vi "Update Message.vi"(8 "error in (no error)":errorcluster, 10 "Message":string, 11 "Chat Room Controller in":refnum<class "Chat Room Controller.lvclass">) -> (0 "error out":errorcluster, 3 "Chat Room Controller out":refnum<class "Chat Room Controller.lvclass">)   [LabVIEW 2018, in "Chat Room Controller.lvlib" / "Chat Room Controller.lvclass"]
uses:
  Chat Room Controller.lvclass
  Chat Room Controller.lvclass/Chat Room Controller.ctl
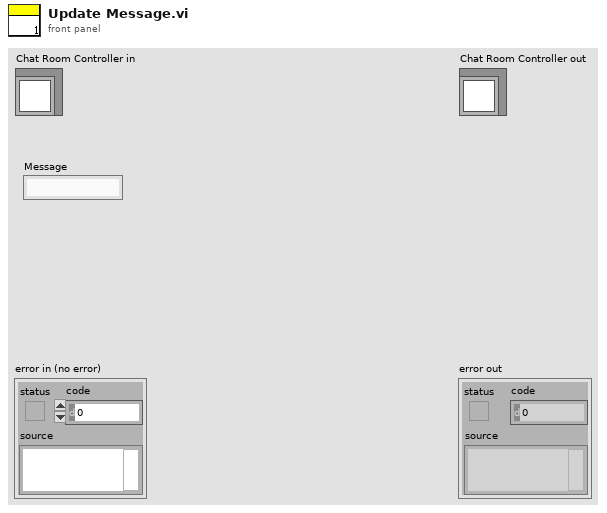
[diagram p1: front panel]
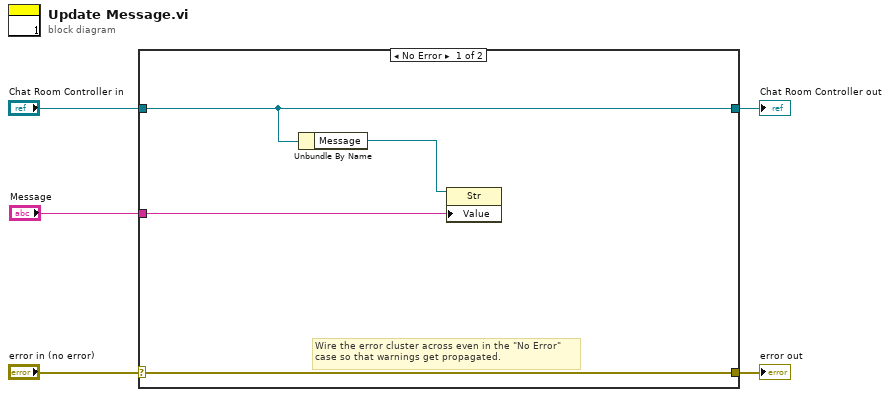
[diagram p0: block diagram]
diagram:
  n1 = case shown="No Error" "error in (no error)" {
    selector: "error in (no error)" -> [w9 w11]
    tunnel: [w9 w11] -> w4
    tunnel: [w8 w10] -> w2
    tunnel: "Chat Room Controller in" -> [w8 w10]
    tunnel: "Message" -> [w6 _]
    frame No Error {
      # "Wire the error cluster across even in the \"No Error\"\ncase so that warnings get propagated."
      n2 = Unbundle By Name(w8) -> ("Message"=w7:refnum<vi>)
      n3 = property class="Str"(reference=w7, "Value"=w6) -> ()  [unwired: 1 in, 2 out]
    }
    frame Error {
    }
  }
  "error out" <- w4
  "Chat Room Controller out" <- w2
